vi "Register for Notification Messages.vi"(8 "error in (no error)":errorcluster, 11 "iCar Position Monitor Model in":refnum<class "iCar Position Monitor Model.lvclass">) -> (0 "error out":errorcluster, 3 "iCar Position Monitor Model out":refnum<class "iCar Position Monitor Model.lvclass">)   [LabVIEW 2019, in "iCar Position Monitor Model.lvclass"]
uses:
  <vilib>/gpm_packages/@cs/Car-wash/Source/iCar Position Monitor Model/iCar Position Monitor Model/iCar Position Monitor Model.lvclass
  C:/Program Files/National Instruments/LabVIEW 2019/vi.lib/gpm_packages/@cs/mva-core/Source/IObserver/IObserver/IObserver.lvclass
  <vilib>/gpm_packages/@cs/Car-wash/Source/iCar Position Monitor Model/iCar Position Monitor Model Messages/Car Position Actual Update Msg/Car Position Actual Update Msg.lvclass
  C:/Program Files/National Instruments/LabVIEW 2019/vi.lib/gpm_packages/@cs/transport/Source/Concrete/ActorMessageTransport/Notification Msg/Notification Msg.lvclass
  <vilib>/gpm_packages/@cs/Car-wash/Source/iCar Position Monitor Model/iCar Position Monitor Model Messages/Car Position Desired Update Msg/Car Position Desired Update Msg.lvclass
  <vilib>/gpm_packages/@cs/mva-core/Source/SubscriptionPolicy/BasicSubscription/BasicSubscription.lvclass/BasicSubscription.ctl
  <vilib>/ActorFramework/Actor/Actor.lvclass/Actor.ctl
  <vilib>/ActorFramework/Message Enqueuer/Message Enqueuer.lvclass/Message Enqueuer.ctl
  <vilib>/gpm_packages/@cs/transport/Source/Concrete/ActorMessageTransport/ActorMessageTransport.lvclass/ActorMessageTransport.ctl
  <vilib>/gpm_packages/@cs/mva-core/Source/IMediator/SubscriptionRequest/SubscriptionRequest.lvclass/SubscriptionRequest.ctl
  <vilib>/gpm_packages/@cs/mva-core/Source/IObserver/IObserver Messages/Subscribe Msg/Subscribe Msg.lvclass/Subscribe Msg.ctl
  <vilib>/gpm_packages/@cs/mva-core/Source/IMediator/SubscriptionRequest/Pack Subscription Request.vi
  <vilib>/gpm_packages/@cs/mva-core/Source/IObserver/IObserver Messages/Subscribe Msg/Send Subscribe.vi
  <vilib>/ActorFramework/Actor/Read Self Enqueuer.vi
  <vilib>/gpm_packages/@cs/transport/Source/Concrete/ActorMessageTransport/Construct Actor Message Transport.vi
  <vilib>/ActorFramework/Message Enqueuer/Enqueue.vi
  <vilib>/ActorFramework/Message Enqueuer/Init from Existing Queue.vi
  <vilib>/ActorFramework/Message Enqueuer/Equals Not A Refnum.vi
  <vilib>/gpm_packages/@cs/mva-core/Source/SubscriptionPolicy/BasicSubscription/BasicSubscription.lvclass
  C:/Program Files/National Instruments/LabVIEW 2019/vi.lib/gpm_packages/@cs/mva-core/Source/IMediator/ISubscriptionPolicy/ISubscriptionPolicy.lvclass
  <vilib>/gpm_packages/@cs/mva-core/Source/IObserver/IObserver/IObserver.lvclass
  C:/Program Files/National Instruments/LabVIEW 2019/vi.lib/ActorFramework/Actor/Actor.lvclass
  <vilib>/gpm_packages/@cs/transport/Source/Concrete/ActorMessageTransport/ActorMessageTransport.lvclass
  C:/Program Files/National Instruments/LabVIEW 2019/vi.lib/gpm_packages/@cs/transport/Source/ITransport/ITransport.lvclass
  <vilib>/gpm_packages/@cs/mva-core/Source/IObserver/IObserver Messages/Subscribe Msg/Subscribe Msg.lvclass
  C:/Program Files/National Instruments/LabVIEW 2019/vi.lib/ActorFramework/Message/Message.lvclass
  <vilib>/Utility/error.llb/Error Cluster From Error Code.vi
  <vilib>/gpm_packages/@cs/mva-core/Source/IMediator/ISubscriptionPolicy/Open Subscription Policy.vi
  <vilib>/ActorFramework/Message Priority Queue/Priority Enqueue.vi
  <vilib>/ActorFramework/Message Enqueuer/Message Enqueuer.lvclass
  <vilib>/gpm_packages/@cs/mva-core/Source/IMediator/SubscriptionRequest/SubscriptionRequest.lvclass
  <vilib>/gpm_packages/@cs/transport/Source/Concrete/ActorMessageTransport/Notification Msg/Notification Msg.lvclass
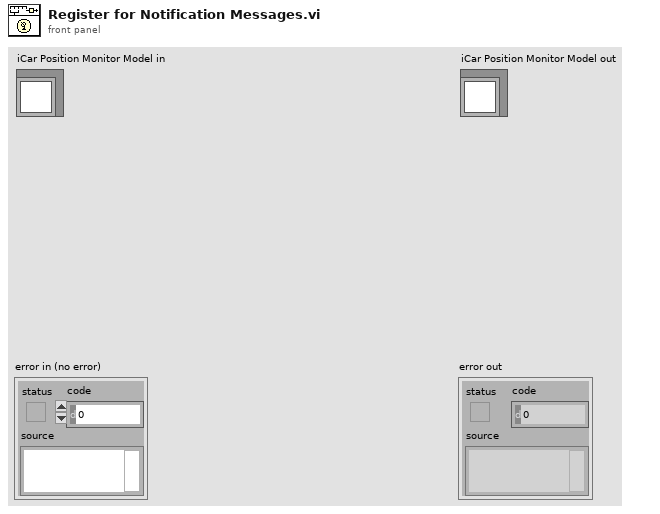
[diagram p1: front panel]
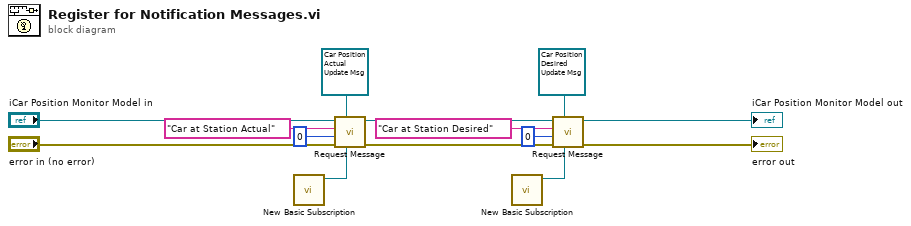
[diagram p0: block diagram]
diagram:
  n1 = call <vilib>:"New Basic Subscription.vi"() -> ("BasicSubscription Out"=w9:refnum<class "BasicSubscription.lvclass">)  [unwired: 11 in]
  n2 = call <vilib>:"Request Message.vi"("Configured SubscriptionPolicy"=w9, "Desired Notification Msg"=refnum<class "Car Position Actual Update Msg.lvclass"> refnum ("Car Position Actual Update Msg.lvclass"), "error in (no error)"="error in (no error)", "Data Type"=u8 0, "Datum Name"="Car at Station Actual", "IObserver in"="iCar Position Monitor Model in") -> ("error out"=w3:errorcluster, "IObserver out"=w5:refnum<class "iCar Position Monitor Model.lvclass">)  [unwired: 3 in, 1 out]
  n3 = call <vilib>:"New Basic Subscription.vi"() -> ("BasicSubscription Out"=w8:refnum<class "BasicSubscription.lvclass">)  [unwired: 11 in]
  n4 = call <vilib>:"Request Message.vi"("Configured SubscriptionPolicy"=w8, "Desired Notification Msg"=refnum<class "Car Position Desired Update Msg.lvclass"> refnum ("Car Position Desired Update Msg.lvclass"), "error in (no error)"=w3, "Data Type"=u8 0, "Datum Name"="Car at Station Desired", "IObserver in"=w5) -> ("error out"=→"error out":errorcluster, "IObserver out"=→"iCar Position Monitor Model out":refnum<class "iCar Position Monitor Model.lvclass">)  [unwired: 3 in, 1 out]
